vi "Set Bias Voltage.vi"(8 "error in (no error)":errorcluster, 9 "Channel":i32, 10 "Bias Voltage (V)":dbl, 11 "Instrument.sample-registry":refnum<class "Instrument.sample-registry.lvclass">) -> (0 "error out":errorcluster, 3 "Instrument.sample-registry out":refnum<class "Instrument.sample-registry.lvclass">)   [LabVIEW 2019, in "Instrument.sample-registry.lvclass"]
uses:
  Instrument.sample-registry.lvclass
  Typedefs/Instrument.sample-registry.Commands--Enum.ctl
  67792bfe-8e2c-4879-abc2-cb448bcec168.vi
  67792bfe-8e2c-4879-abc2-cb448bcec168.vi/c75e12d4-2661-49a5-9afc-dbffdb694870.vi
  67792bfe-8e2c-4879-abc2-cb448bcec168.vi/2a0bf3c4-890a-488b-bba9-7d0e50155bd9.vi
  67792bfe-8e2c-4879-abc2-cb448bcec168.vi/2a0bf3c4-890a-488b-bba9-7d0e50155bd9.vi/a640b9e0-2bb1-42d0-9491-26b19c1d8e7b.vi
  67792bfe-8e2c-4879-abc2-cb448bcec168.vi/2a0bf3c4-890a-488b-bba9-7d0e50155bd9.vi/8610e4ee-7e05-4c89-86eb-49a2000bc7ea.vi
  <userlib>/LevyLab/Levylab Instruments/SMOs/RemoteControl/API/Remote Client.vi
  <vilib>/JDP Science/JSONtext/JSON text to Variant.vi
  <vilib>/JDP Science/JSONtext/LVClass Serializer/JSONtext LVClass Serializer.lvclass
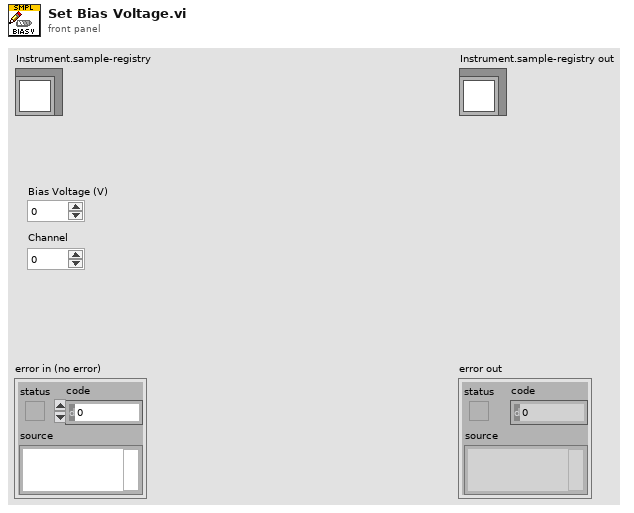
[diagram p1: front panel]
types:
  T1 = typedef "Instrument.sample-registry.lvclass/Instrument.sample-registry.Commands--Enum.ctl" = enum16{"Set User", "Get User", "Set Sample", "Get Sample"}
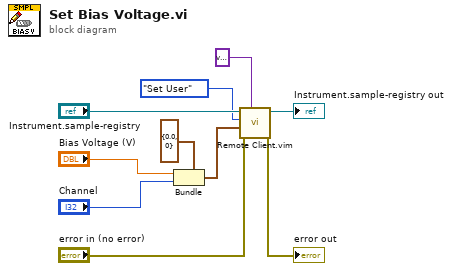
[diagram p0: block diagram]
diagram:
  n1 = Bundle(cluster=cluster{"Bias Voltage (V)":dbl, "Channel":i32} {"Bias Voltage (V)"=0.0, "Channel"=0} ("output cluster"), "Bias Voltage (V)"="Bias Voltage (V)", "Channel"="Channel") -> (w3:cluster{"Bias Voltage (V)":dbl, "Channel":i32})
  n2 = call "Remote Client.vim"("Data Out type"=variant, "error in (no error)"="error in (no error)", "params"=w3, "method"=Instrument.sample-registry.Commands--Enum."Set User" ("Commands"), "Instrument in"="Instrument.sample-registry") -> ("error out"=→"error out":errorcluster, "Instrument out"=→"Instrument.sample-registry out":refnum<class "Instrument.sample-registry.lvclass">)  [unwired: 3 in, 2 out]
